vi "responder action.vi"(10 "dictionary":variant, 11 "standard input":string) -> (1 "code":u32, 2 "standard error":string, 3 "standard out":string)   [LabVIEW 2013]
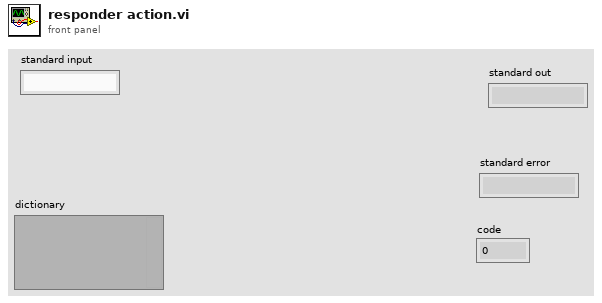
[diagram p1: front panel]
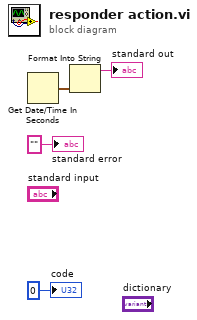
[diagram p0: block diagram]
diagram:
  n1 = Get Date/Time In Seconds() -> (seconds since 1Jan1904=w1:timestamp)
  n2 = Format Into String(w1) -> (resulting string=→"standard out":string)  [unwired: 3 in, 1 out]
  "standard error" <- "" ("standard error")
  "code" <- u32 0 ("code")
